vi "NI change z offset.vi"(8 "error in (no error)":errorcluster, 10 "offset":dbl, 11 "NI in":refnum<class "NI.lvclass">) -> (0 "error out":errorcluster, 3 "NI out":refnum<class "NI.lvclass">)   [LabVIEW 2021, in "NI.lvlib" / "NI.lvclass"]
uses:
  NI.lvclass
  NI.lvclass/NI.ctl
  <vilib>/DAQmx/write.llb/DAQmx Write (Analog 2D DBL NChan NSamp).vi
  <vilib>/DAQmx/miscellaneous.llb/DAQmx Fill In Error Info.vi
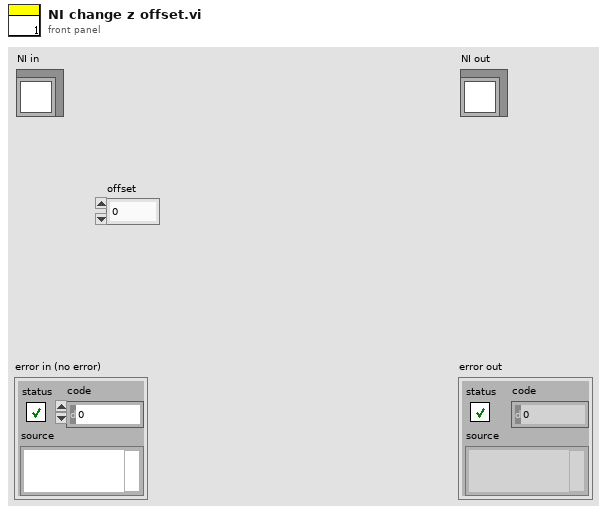
[diagram p1: front panel]
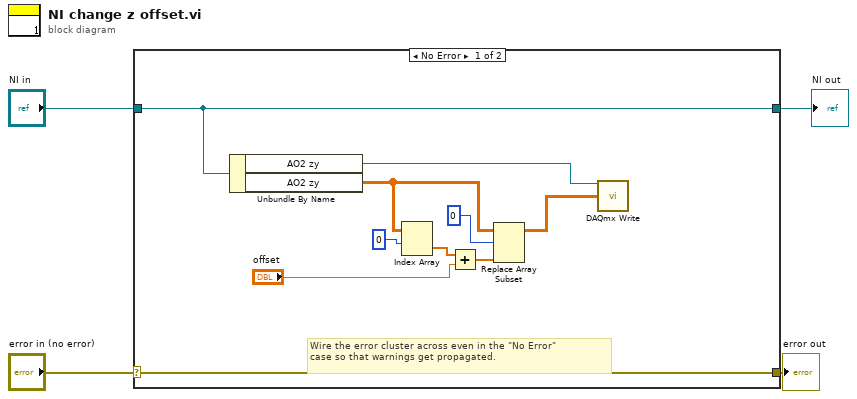
[diagram p0: block diagram]
diagram:
  n1 = case shown="No Error" "error in (no error)" {
    selector: "error in (no error)" -> [w14 w16]
    tunnel: [w14 w16] -> w3
    tunnel: [w13 w15] -> w1
    tunnel: "NI in" -> [w13 w15]
    frame No Error {
      # "Wire the error cluster across even in the \"No Error\"\ncase so that warnings get propagated."
      n2 = Unbundle By Name(w13) -> ("AO2 zy"=w7:refnum<k21>, "AO2 zy"=w8:dbl[][])
      n3 = Index Array(array=w8, index (row)=0) -> (element=w11:dbl[])  [unwired: 1 in]
      n4 = Add(x=w11, y="offset") -> (x+y=w12:dbl[])
      n5 = Replace Array Subset(array=w8, new element=w12, index (row)=0) -> (w6:dbl[][])  [unwired: 1 in]
      n6 = call-poly <vilib>:"DAQmx Write.vi"("task/channels in"=w7, "data"=w6) -> ()  [unwired: 11 in, 3 out]
    }
    frame Error {
    }
  }
  "error out" <- w3
  "NI out" <- w1
